vi "Set Async Processing Rates.vi"(8 "error in":errorcluster, 9 "Outgoing Frame Rate":dbl caption="Outgoing frame processing rate [Hz]" min=0.0, 10 "Incoming Frame Rate":dbl caption="Incoming frame processing rate [Hz]" min=0.0, 11 "custom device ref":T1 format="%.0x") -> (0 "error out":errorcluster, 3 "custom device ref out":T1 format="%.0x")   [LabVIEW 2020, in "AIM ARINC 664 Scripting.lvlib"]
uses:
  AIM ARINC 664 Scripting.lvlib
  <vilib>/NI VeriStand/Custom Device API/Custom Device API.lvlib
  Constants.vi
  <vilib>/NI VeriStand/Custom Device API/Set Item Property (Double).vi
  <vilib>/NI VeriStand/Custom Device API/Custom Device Item Ref.ctl
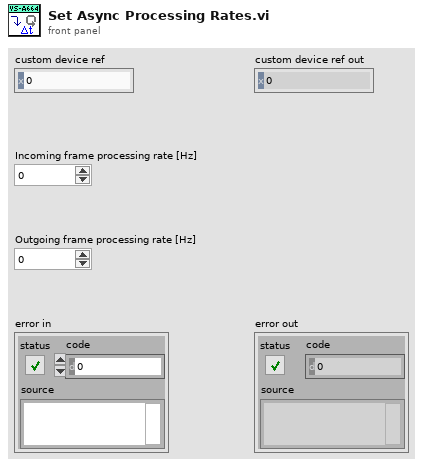
[diagram p1: front panel]
types:
  T1 = typedef "Custom Device API.lvlib/Custom Device Item Ref.ctl" = u64
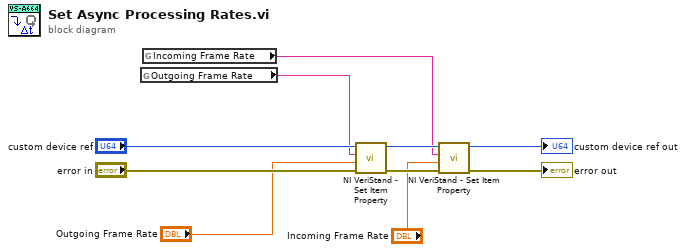
[diagram p0: block diagram]
diagram:
  n1 = global read "Constants.vi" "Outgoing Frame Rate"() -> (w4:string)
  n2 = global read "Constants.vi" "Incoming Frame Rate"() -> (w3:string)
  n3 = call-poly <vilib>:"NI VeriStand - Set Item Property.vi"("error in (no error)"="error in", "Value"="Outgoing Frame Rate", "Property Name"=w4, "Item Ref in"="custom device ref") -> ("error out"=w6:errorcluster, "Item Ref out"=w9:T1)  [unwired: 5 in, 1 out]
  n4 = call-poly <vilib>:"NI VeriStand - Set Item Property.vi"("error in (no error)"=w6, "Value"="Incoming Frame Rate", "Property Name"=w3, "Item Ref in"=w9) -> ("error out"=→"error out":errorcluster, "Item Ref out"=→"custom device ref out":T1)  [unwired: 5 in, 1 out]
